vi "Get Siblings.vi"(8 "error in (no error)":errorcluster, 10 "Tag":string, 11 "Tree in":refnum<class "TreeControl.lvclass">) -> (0 "error out":errorcluster, 2 "SiblingTags[]":string[](array[string]), 3 "Tree out":refnum<class "TreeControl.lvclass">)   [LabVIEW 2015, in "TreeControl.lvclass"]
doc: "This method returns an array of the siblings (items on the same level and having the same parent) of the given item, including itself.\n<b> </b> <b> </b>\n©2016 Q Software Innovations, LLC (QSI)\nwritten by Quentin Alldredge\nproduced in LabVIEW 2015\n\nsupport@qsoftwareinnovations.com\nwww.qsoftwareinnovations.com\n\nAll rights reserved.\n\nRedistribution and use in source and binary forms, with or without modification, are permitted provided that the following conditions are met:\n\n * Redistributions of source code must retain the above copyright notice, this list of conditions and the following disclaimer.\n * Redistributions in binary form must reproduce the above copyright notice, this list of conditions and the following disclaimer in the documentation and/or other materials provided with the distribution.\n * Neither the name of Q Software Innovations, LLC. nor the names of its contributors may be used to endorse or promote products derived from this software without specific prior written permission.\n\nTHIS SOFTWARE IS PROVIDED BY THE COPYRIGHT HOLDERS AND CONTRIBUTORS \"AS IS\" AND ANY EXPRESS OR IMPLIED WARRANTIES, INCLUDING, BUT NOT LIMITED TO, THE IMPLIED WARRANTIES OF MERCHANTABILITY AND FITNESS FOR A PARTICULAR PURPOSE ARE DISCLAIMED. IN NO EVENT SHALL THE COPYRIGHT OWNER OR CONTRIBUTORS BE LIABLE FOR ANY DIRECT, INDIRECT, INCIDENTAL, SPECIAL, EXEMPLARY, OR CONSEQUENTIAL DAMAGES (INCLUDING, BUT NOT LIMITED TO, PROCUREMENT OF SUBSTITUTE GOODS OR SERVICES; LOSS OF USE, DATA, OR PROFITS; OR BUSINESS INTERRUPTION) HOWEVER CAUSED AND ON ANY THEORY OF LIABILITY, WHETHER IN CONTRACT, STRICT LIABILITY, OR TORT (INCLUDING NEGLIGENCE OR OTHERWISE) ARISING IN ANY WAY OUT OF THE USE OF THIS SOFTWARE, EVEN IF ADVISED OF THE POSSIBILITY OF SUCH DAMAGE."
uses:
  TreeControl.lvclass
  TreeControl.lvclass/TreeControl.ctl
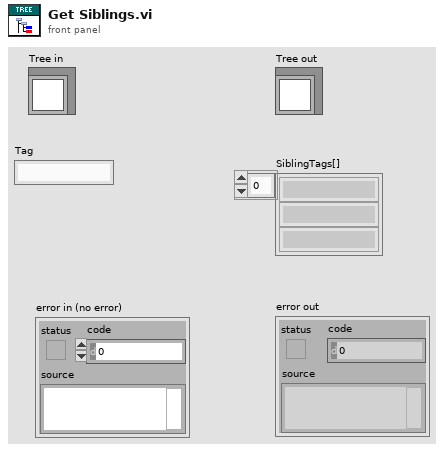
[diagram p1: front panel]
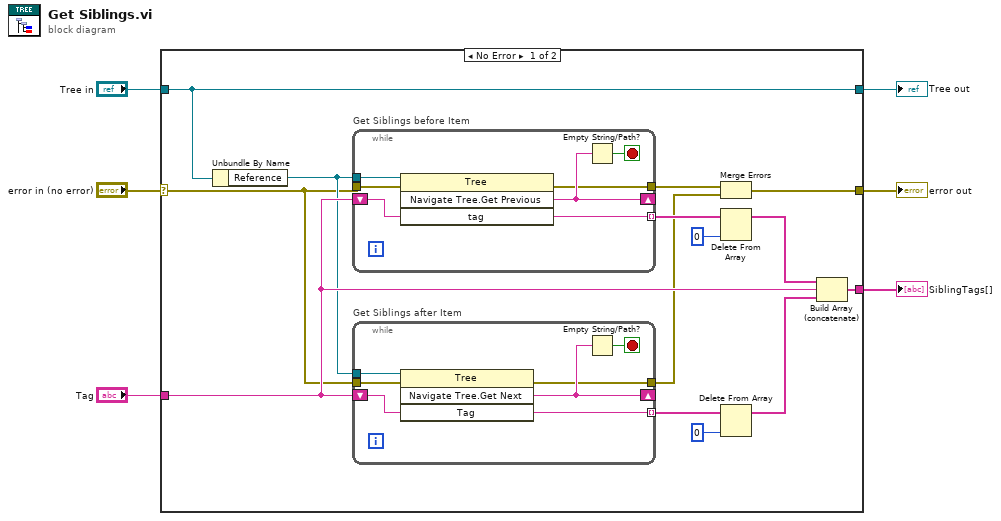
[diagram p0: block diagram]
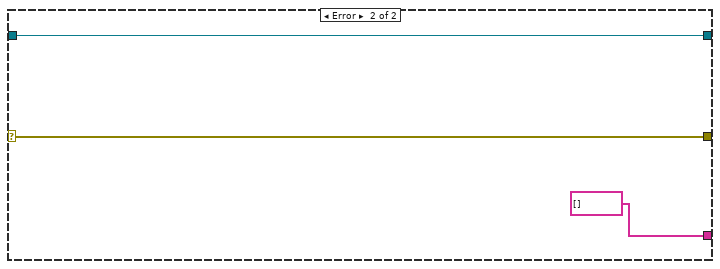
[diagram p2: hidden frame]
diagram:
  n1 = case shown="No Error" "error in (no error)" {
    selector: "error in (no error)" -> [w7 w35]
    tunnel: "Tag" -> [w16 _]
    tunnel: [w13 string[] []] -> w5
    tunnel: [w10 w35] -> w3
    tunnel: "Tree in" -> [w9 w33]
    tunnel: [w9 w33] -> w1
    frame No Error {
      n2 = Unbundle By Name(w9) -> ("Reference"=w8:refnum<vi>)
      n3 = while "Get Siblings before Item" {
        tunnel: w8 -> [w32]
        shift-right: [w30] -> _
        shift-left: w16 -> [w31]
        tunnel: [w31] -> w20 mode=indexing
        tunnel: [w28] -> w12
        tunnel: w7 -> [w27]
        stop <- w29 stop-if-true
        n4 = invoke class="Tree" method="Navigate Tree.Get Previous"(reference=w32, error in=w27, "tag"=w31) -> (error out=w28:errorcluster, "Navigate Tree:Get Previous"=w30:string)  [unwired: 1 in, 2 out]
        n5 = Empty String/Path?(string/path=w30) -> (empty?=w29:bool)
      }
      n6 = while "Get Siblings after Item" {
        tunnel: w8 -> [w26]
        shift-right: [w24] -> _
        shift-left: w16 -> [w25]
        tunnel: [w25] -> w19 mode=indexing
        tunnel: [w22] -> w11
        tunnel: w7 -> [w21]
        stop <- w23 stop-if-true
        n7 = invoke class="Tree" method="Navigate Tree.Get Next"(reference=w26, error in=w21, "Tag"=w25) -> (error out=w22:errorcluster, "Navigate Tree:Get Next Item"=w24:string)  [unwired: 1 in, 2 out]
        n8 = Empty String/Path?(string/path=w24) -> (empty?=w23:bool)
      }
      n9 = Merge Errors(w12, w11) -> (w10:errorcluster)
      n10 = Delete From Array(array=w20, index=0) -> (array with subset deleted=w15:string[])  [unwired: 1 in, 1 out]
      n11 = Delete From Array(array=w19, index=0) -> (array with subset deleted=w14:string[])  [unwired: 1 in, 1 out]
      n12 = Build Array (concatenate)(w15, w16, w14) -> (w13:string[])
    }
    frame Error {
    }
  }
  "SiblingTags[]" <- w5
  "error out" <- w3
  "Tree out" <- w1
